vi "Convert_StringToU8Array.vi"(9 "text array":string[](array[string])) -> (1 "U8 array":u8[](array[numeric]))   [LabVIEW 2010, in "Pansino_XML_Read.lvlib"]
uses:
  Pansino_XML_Read.lvlib
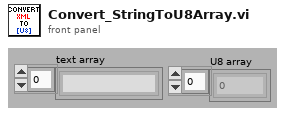
[diagram p1: front panel]
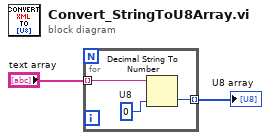
[diagram p0: block diagram]
diagram:
  n1 = for {
    tunnel: "text array" -> [w3] mode=indexing
    tunnel: [w5] -> w1 mode=indexing
    w4 = u8 0  # U8
    n2 = Decimal String To Number(string=w3, default (0L)=w4) -> (number=w5:u8)  [unwired: 1 in, 1 out]
  }
  "U8 array" <- w1
